vi "StopWatch_Panel.vi"() -> ()   [LabVIEW 2025]
panel:
  in  "?":enum32{"Page 1", "Page 2"}(tab)
  in  "Reset":bool
  in  "Start":bool
  out "Second":dbl
  out "Minute":dbl
  out "Hour":dbl
  out "?":bool
  # "Digital Stop Watch"
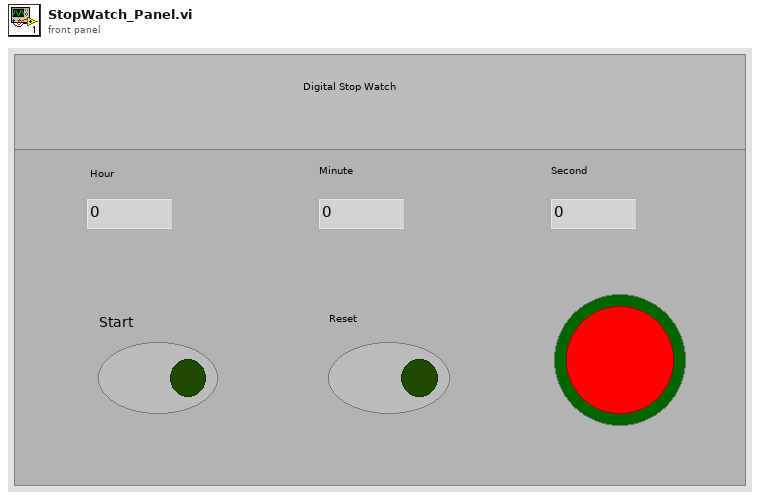
[diagram p1: front panel]
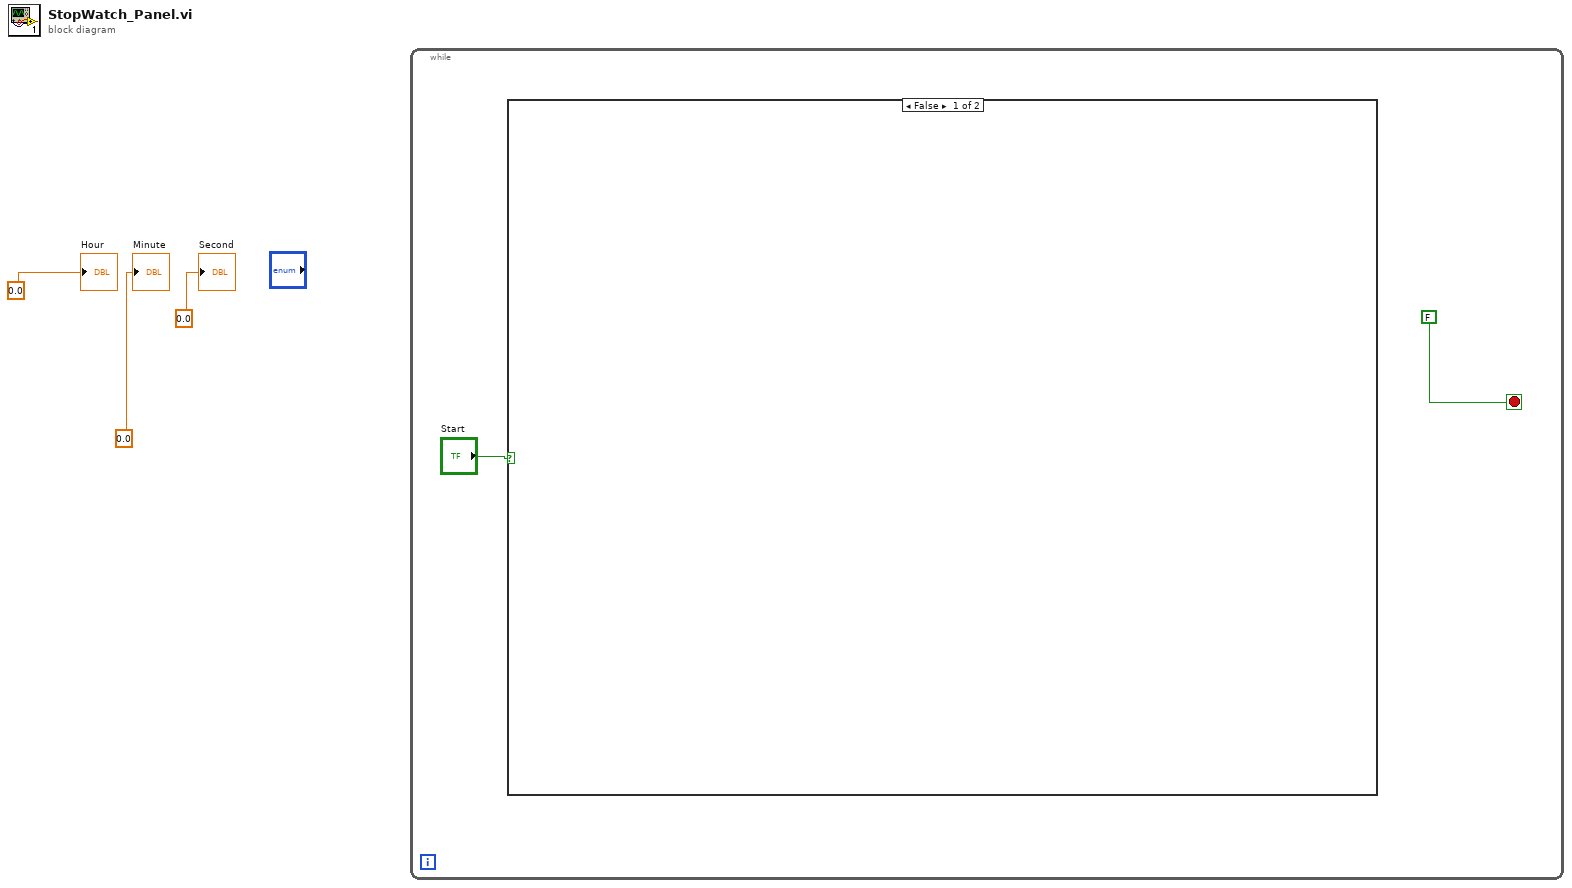
[diagram p0: block diagram]
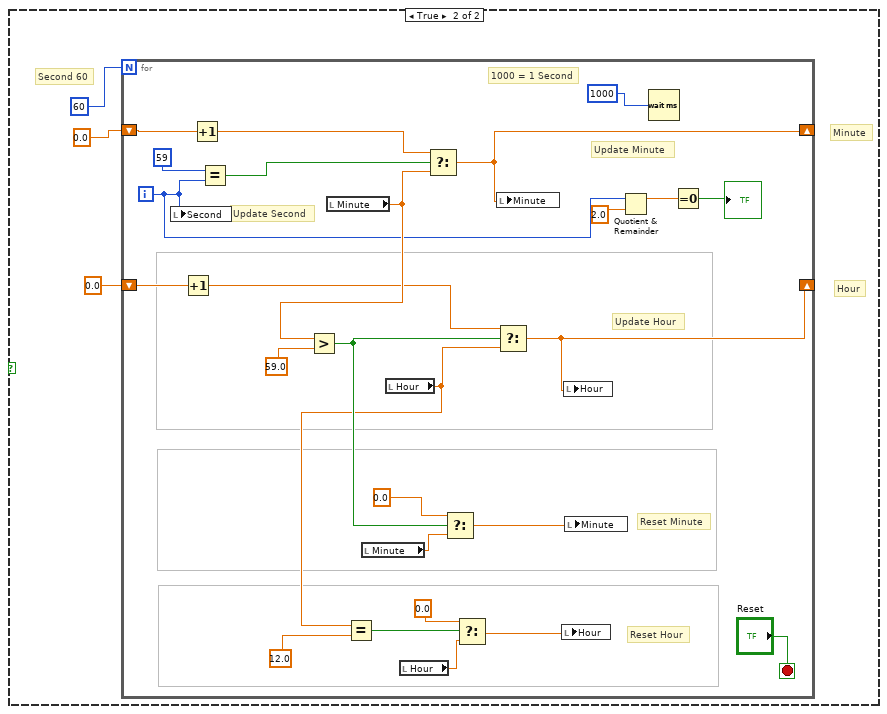
[diagram p2: hidden frame]
diagram:
  n1 = while {
    stop <- FALSE ("Stop") stop-if-true
    n2 = case shown="False" "Start" {
      frame False {
      }
      frame True {
        # "Hour"
        # "Minute"
        # "Second 60"
        n3 = for {
          N: 60 -> [_]
          shift-right: [w30] -> _
          shift-left: 0.0 -> [w32]
          shift-right: [w15] -> _
          shift-left: 0.0 ("Hr") -> [w29]
          i -> [w9]
          stop <- "Reset" stop-if-true
          # "Update Second"
          # "Update Minute"
          # "Update Hour"
          # "Reset Minute"
          # "Reset Hour"
          # "1000 = 1 Second"
          n4 = local write "Second"(w9) -> ()
          n5 = Increment(x=w29) -> (x+1=w26:dbl)
          n6 = Increment(x=w32) -> (x+1=w31:dbl)
          n7 = Equal?(x=59, y=w9) -> (x = y?=w33:bool)
          n8 = local read "Minute"() -> (w28:dbl)
          n9 = Greater?(x=w28, y=59.0) -> (0:w24:bool)
          n10 = local read "Minute"() -> (w23:dbl)
          n11 = local read "Hour"() -> (w14:dbl)
          n12 = Equal?(x=w14, y=12.0) -> (x = y?=w20:bool)
          n13 = local read "Hour"() -> (w19:dbl)
          n14 = Select(t=w31, s=w33, f=w28) -> (s? t:f=w30:dbl)
          n15 = Select(t=0.0, s=w24, f=w23) -> (s? t:f=w22:dbl)
          n16 = Select(t=0.0, s=w20, f=w19) -> (s? t:f=w17:dbl)
          n17 = local write "Minute"(w30) -> ()
          n18 = Select(t=w26, s=w24, f=w14) -> (s? t:f=w15:dbl)
          n19 = local write "Hour"(w17) -> ()
          n20 = local write "Hour"(w15) -> ()
          n21 = local write "Minute"(w22) -> ()
          n22 = Quotient & Remainder(x=w9, y=2.0) -> (x-y*floor(x/y)=w12:dbl)  [unwired: 1 out]
          n23 = Wait (ms)(milliseconds to wait=u32 1000) -> ()  [unwired: 1 out]
          n24 = Equal To 0?(x=w12) -> (x = 0?=→"?":bool)
        }
      }
    }
  }
  "Hour" <- 0.0 ("Hr")
  "Minute" <- 0.0 ("Min")
  "Second" <- 0.0 ("Sec")
